vi "FVIR_LDO_Ultramat_23.vi"(8 "error in":errorcluster, 10 "VISA resource name":refnum<visa-resource-name>="OXYMAT", 11 "Message Queues":T1) -> (0 "error out":errorcluster)   [LabVIEW 2020]
uses:
  Message Queue/All Message Queues.ctl
  Message Queue/Message Cluster.ctl
  Message Queue/Enqueue Message (Single).vi
  Message Queue/Message Queue.lvlib
panel:
  out "Gas Type":string
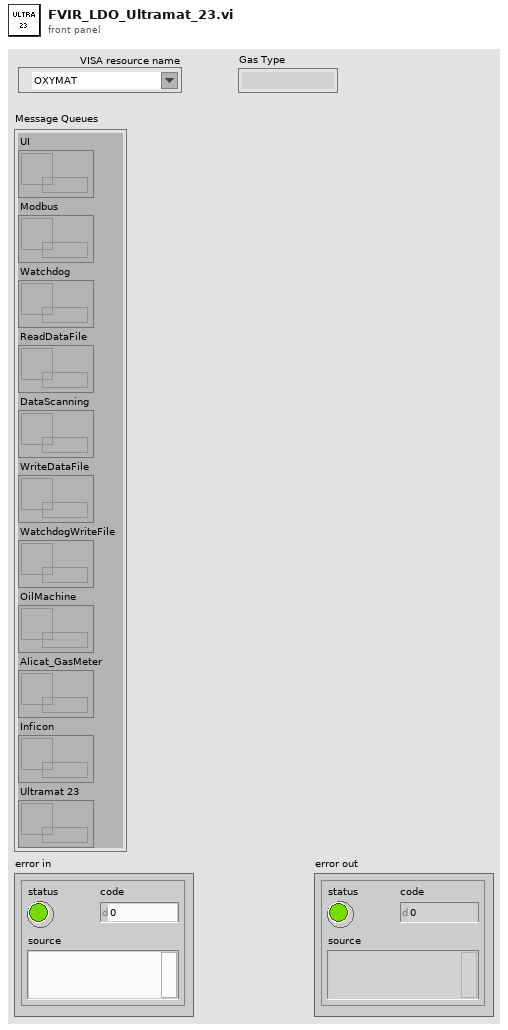
[diagram p1: front panel]
types:
  T1 = typedef "Message Queue.lvlib/All Message Queues.ctl" = cluster{"UI":refnum<queue>, "Modbus":refnum<queue>, "Watchdog":refnum<queue>, "ReadDataFile":refnum<queue>, "DataScanning":refnum<queue>, "WriteDataFile":refnum<queue>, "WatchdogWriteFile":refnum<queue>, "OilMachine":refnum<queue>, "Alicat_GasMeter":refnum<queue>, "Inficon":refnum<queue>, "Ultramat 23":refnum<queue>}
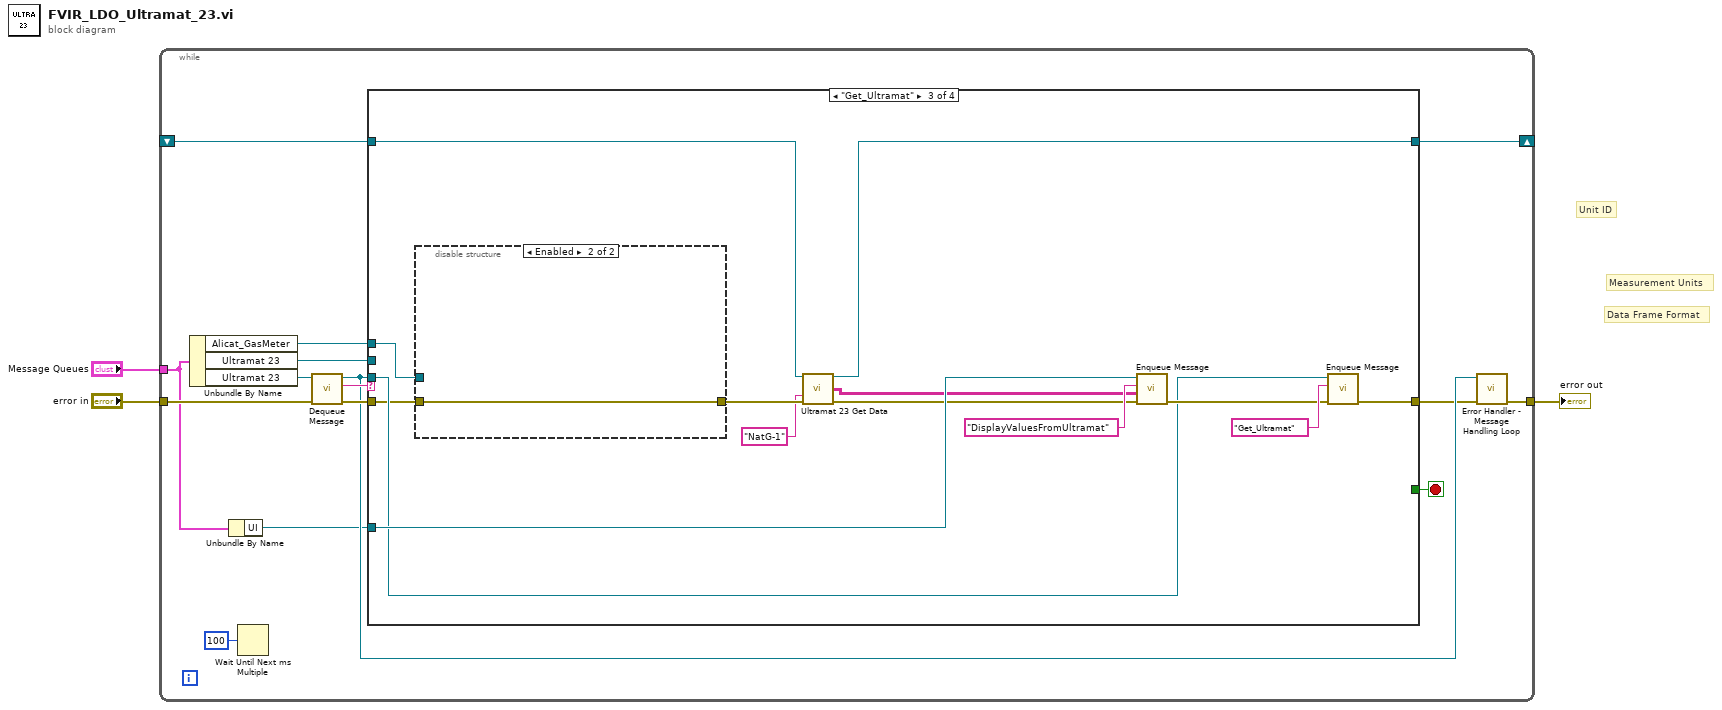
[diagram p0: block diagram]
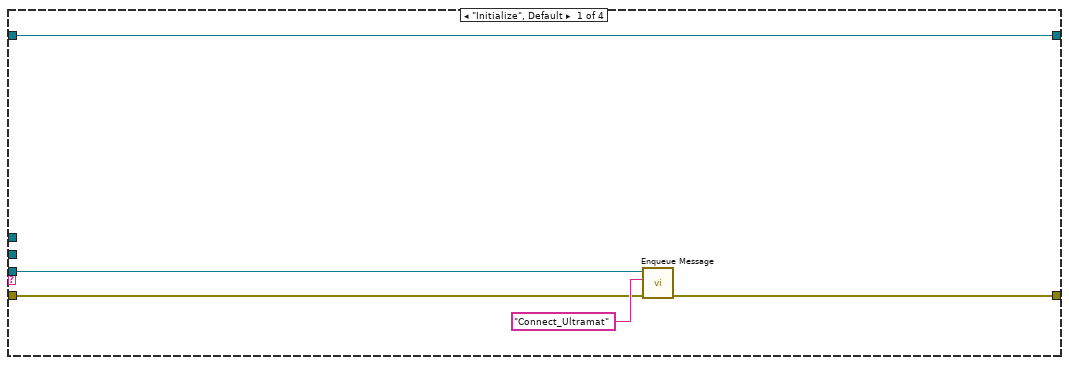
[diagram p2: hidden frame]
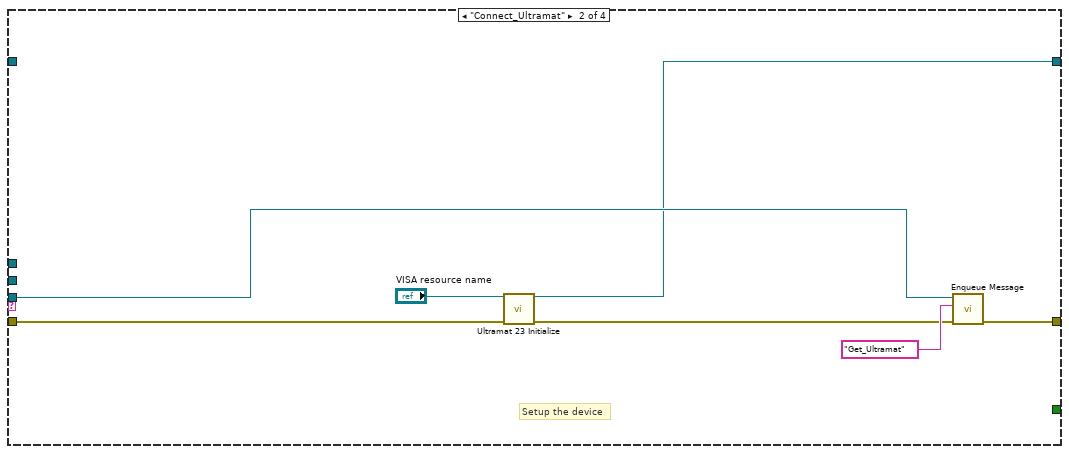
[diagram p3: hidden frame]
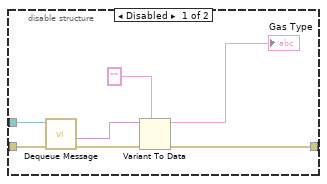
[diagram p4: hidden frame]
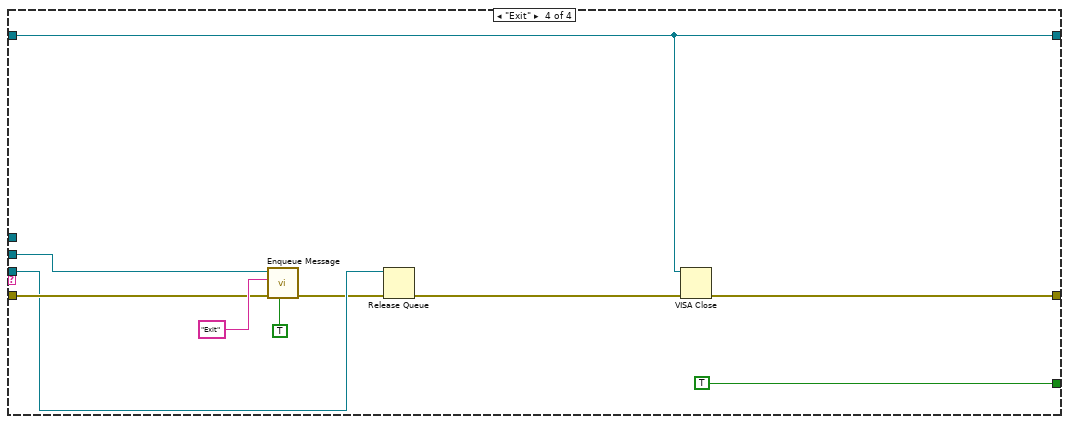
[diagram p5: hidden frame]
diagram:
  # "Unit ID"
  # "Data Frame Format"
  # "Measurement Units"
  n1 = while {
    tunnel: "Message Queues" -> [w8]
    tunnel: "error in" -> [w17]
    tunnel: [w11] -> w1
    shift-right: [w6] -> _
    shift-left: _ -> [w5]
    stop <- w14 stop-if-true
    n2 = Unbundle By Name(w8) -> ("Alicat_GasMeter"=w4:refnum<queue>, "Ultramat 23"=w13:refnum<queue>, "Ultramat 23"=w18:refnum<queue>)
    n3 = Unbundle By Name(w8) -> ("UI"=w7:refnum<queue>)
    n4 = Wait Until Next ms Multiple(millisecond multiple=u32 100) -> ()  [unwired: 1 out]
    n5 = call "Dequeue Message.vi"("error in (no error)"=w17, "Message Queue"=w18) -> ("error out"=w15:errorcluster, "Message"=w16:string, "dup Message Queue"=w12:refnum<queue>)  [unwired: 6 in, 1 out]
    n6 = case shown="\"Get_Ultramat\"" w16 {
      tunnel: w15 -> [w22 w27 w34 w58]
      tunnel: [w21 w29 w40 w54] -> w10
      tunnel: [_ _ _ TRUE] -> w14
      tunnel: w13 -> [_ _ _ w59]
      tunnel: w12 -> [w20 w28 w39 w57]
      tunnel: w7 -> [_ _ w43 _]
      tunnel: [w19 w24 w36 w53] -> w6
      tunnel: w5 -> [w19 _ w37 w53]
      tunnel: w4 -> [_ _ w33 _]
      frame "Initialize", Default {
        n7 = call-poly "Enqueue Message.vi"("error in (no error)"=w22, "Message"="Connect_Ultramat", "Message Queue"=w20) -> ("error out"=w21:errorcluster)  [unwired: 7 in, 1 out]
      }
      frame "Connect_Ultramat" {
        # "Setup the device"
        n8 = call "Ultramat 23 Initialize.vi"("VISA resource name"="VISA resource name", "error in (no error)"=w27) -> ("VISA Session Out"=w24:refnum<visa-resource-name>, "error out"=w26:errorcluster)  [unwired: 8 in, 4 out]
        n9 = call-poly "Enqueue Message.vi"("error in (no error)"=w26, "Message"="Get_Ultramat", "Message Queue"=w28) -> ("error out"=w29:errorcluster)  [unwired: 7 in, 1 out]
      }
      frame "Get_Ultramat" {
        n10 = disable-structure shown="Enabled" {
          disable-tunnel: w34 -> [w51 w52]
          disable-tunnel: w33 -> [w50 _]
          disable-tunnel: [w46 w52] -> w32
          frame Disabled {
            n11 = call "Dequeue Message.vi"("error in (no error)"=w51, "Message Queue"=w50) -> ("error out"=w49:errorcluster, "Message Data"=w47:variant)  [unwired: 6 in, 2 out]
            n12 = Variant To Data(error in=w49, type="", Variant=w47) -> (data=→"Gas Type":string, error out=w46:errorcluster)
          }
          frame Enabled {
          }
        }
        n13 = call "Ultramat 23 Get Data.vi"("VISA resource name"=w37, "Gas selected"="NatG-1", "error in (no error)"=w32) -> ("VISA Session Out"=w36:refnum<visa-resource-name>, "Data Array"=w35:string[][], "error out"=w38:errorcluster)  [unwired: 8 in, 2 out]
        n14 = call-poly "Enqueue Message.vi"("error in (no error)"=w38, "Message Data"=w35, "Message"="DisplayValuesFromUltramat", "Message Queue"=w43) -> ("error out"=w41:errorcluster)  [unwired: 6 in, 1 out]
        n15 = call-poly "Enqueue Message.vi"("error in (no error)"=w41, "Message"="Get_Ultramat", "Message Queue"=w39) -> ("error out"=w40:errorcluster)  [unwired: 7 in, 1 out]
      }
      frame "Exit" {
        n16 = call-poly "Enqueue Message.vi"("Priority Message? (F)"=TRUE, "error in (no error)"=w58, "Message"="Exit", "Message Queue"=w59) -> ("error out"=w56:errorcluster)  [unwired: 6 in, 1 out]
        n17 = Release Queue(queue=w57, error in (no error)=w56) -> (error out=w55:errorcluster)  [unwired: 1 in, 2 out]
        n18 = VISA Close(VISA resource name=w53, error in (no error)=w55) -> (error out=w54:errorcluster)
      }
    }
    n19 = call "Error Handler - Message Handling Loop.vi"("error in (no error)"=w10, "Message Queue"=w12) -> ("dup error in"=w11:errorcluster)  [unwired: 8 in, 1 out]
  }
  "error out" <- w1
